vi "HandleFileSize.vi"(0 "FName Increment Count":u8, 1 "path":path, 5 "Save Type":u16(ring)=1 items=["USB", "cRIO"], 7 "Filename":string, 9 "Bin Header":i32, 11 "error in":errorcluster, 12 "Max File Size (MB)":i64=500) -> (3 "Low on Free Disk Space":bool, 4 "Current Free Space (Mb)":dbl, 6 "New Save Type":u16, 8 "New Fname":string, 10 "NewFnameCount":u8, 14 "NewFileName Check":bool, 15 "error out":errorcluster)   [LabVIEW 2015]
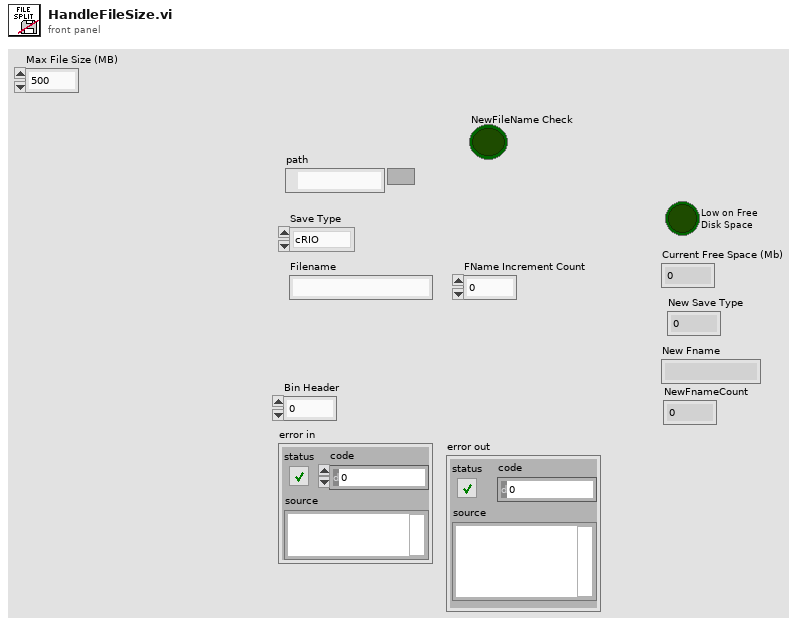
[diagram p1: front panel]
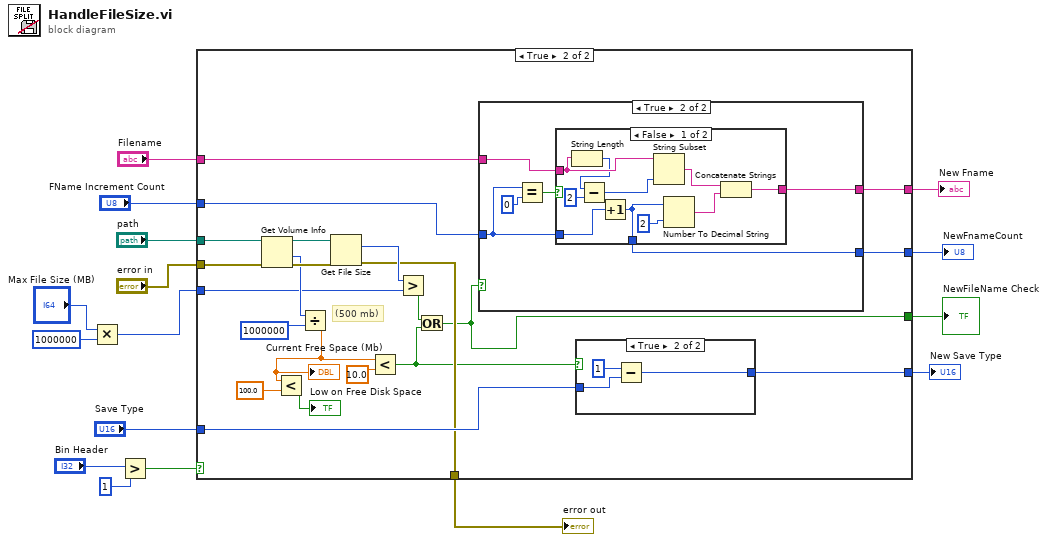
[diagram p0: block diagram]
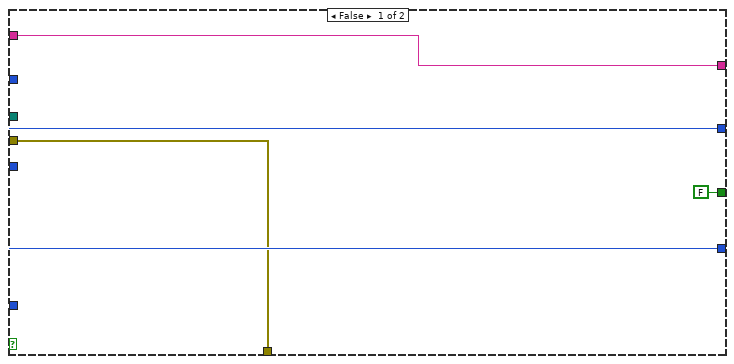
[diagram p2: hidden frame]
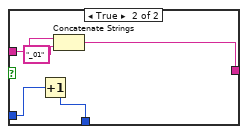
[diagram p4: hidden frame]
diagram:
  n1 = Multiply(x="Max File Size (MB)", y=i64 1000000) -> (x*y=w1:i64)
  n2 = Greater?(x="Bin Header", y=1) -> (0:w11:bool)
  n3 = case shown="True" w11 {
    tunnel: "Filename" -> [w20 w43]
    tunnel: "Save Type" -> [w19 w42]
    tunnel: "FName Increment Count" -> [w21 w40]
    tunnel: [w19 w31] -> w10
    tunnel: [w20 w30] -> w9
    tunnel: [w21 w29] -> w8
    tunnel: "path" -> [_ w28]
    tunnel: [w18 w27] -> w6
    tunnel: "error in" -> [w18 w26]
    tunnel: [FALSE w23] -> w4
    tunnel: w1 -> [_ w22]
    frame False {
    }
    frame True {
      # "(500 mb)"
      n4 = Get Volume Info(8:w26, 11:w28) -> (0:w38:errorcluster, 1:w36:i64, 3:w41:path)  [unwired: 3 out]
      n5 = Divide(x=w36, y=i64 1000000) -> (x/y=w33:dbl)
      "Current Free Space (Mb)" <- w33
      n6 = Less?(x=w33, y=100.0) -> (x < y?=→"Low on Free Disk Space":bool)
      n7 = Get File Size(file=w41, error in=w38) -> (size (in bytes)=w37:i64, 0:w27:errorcluster)  [unwired: 1 out]
      n8 = Less?(x=w33, y=10.0) -> (x < y?=w24:bool)
      n9 = Greater?(x=w37, y=w22) -> (0:w25:bool)
      n10 = Or(x=w25, y=w24) -> (x .or. y?=w23:bool)
      n11 = case shown="True" w23 {
        tunnel: w43 -> [w45 w49]
        tunnel: [w45 w48] -> w30
        tunnel: [w44 w47] -> w29
        tunnel: w40 -> [w44 w46]
        frame False {
        }
        frame True {
          n12 = Equal?(x=w46, y=u8 0) -> (x = y?=w50:bool)
          n13 = case shown="False" w50 {
            tunnel: w49 -> [w61 w66]
            tunnel: [w54 w64] -> w47
            tunnel: [w53 w63] -> w48
            tunnel: w46 -> [w52 w62]
            frame False {
              n14 = String Length(string=w61) -> (length=w58:i32)
              n15 = Subtract(x=w58, y=2) -> (x-y=w57:i32)
              n16 = Increment(x=w52) -> (x+1=w54:u8)
              n17 = String Subset(string=w61, length (rest)=w57) -> (substring=w55:string)  [unwired: 1 in]
              n18 = Number To Decimal String(number=w54, width (-)=i16 2) -> (decimal integer string=w56:string)
              n19 = Concatenate Strings(w55, w56) -> (w53:string)
            }
            frame True {
              n20 = Increment(x=w62) -> (x+1=w64:u8)
              n21 = Concatenate Strings(w66, "_01" ("string")) -> (w63:string)
            }
          }
        }
      }
      n22 = case shown="True" w24 {
        tunnel: w42 -> [w67 w69]
        tunnel: [w67 w68] -> w31
        frame False {
        }
        frame True {
          n23 = Subtract(x=u16 1, y=w69) -> (x-y=w68:u16)
        }
      }
    }
  }
  "New Save Type" <- w10
  "NewFnameCount" <- w8
  "New Fname" <- w9
  "error out" <- w6
  "NewFileName Check" <- w4
